vi "Semianalisys.vi"() -> ()   [LabVIEW 2013]
panel:
  in  "?":enum32{"Diode", "BJT", "FET"}(tab)
  out "Voltage versus current curve of diode":cluster{dbl[], dbl[]}(graph)
  out "Ib versus Vbe progress":dbl(slide) scale=0.0..100.0
  in  "R (kOhm)":dbl=1000000.0 format="%#_13g"
  in  "V_AO0 step (V)":dbl=0.01 format="%#_13g"
  in  "OK Button 5":bool
  in  "OK Button":bool
  in  "OK Button 2":bool
  out "Vce versus Ic curve(s)":cluster{"Array":dbl[], dbl[]}(graph)
  out "Ic versus Vce progress":dbl(slide) scale=0.0..100.0
  out "Vbe versus Ib curve":cluster{dbl[], dbl[]}(graph)
  out "Ib versus Vbe progress":dbl(slide) scale=0.0..100.0
  in  "Set several Ib to be plotted on Ic graph (uA)":dbl[](array[numeric])
  in  "Number of curves":i32
  in  "Vce step (V)":dbl=0.1 format="%#_13g"
  in  "R collector (Ohm)":dbl=470.0 format="%#_13g"
  in  "R base (kOhm)":dbl=1000000.0 format="%#_13g"
  in  "Vbe step (V)":dbl=0.01 format="%#_13g"
  in  "Number of curves":i32
  in  "Set several Vgs to be plotted on Vds graph (V)":dbl[](array[numeric])
  in  "Type of FET":u16(ring) items=["JFET", "DMOSFET", "EMOSFET"]
  in  "Vgs step (V)":dbl=0.1 format="%#_13g"
  in  "OK Button 6":bool
  in  "OK Button 7":bool
  in  "R drain (Ohm)":dbl=993.0 format="%#_13g"
  in  "Vds step (V)":dbl=0.1 format="%#_13g"
  out "Id versus Vgs curve":cluster{dbl[], dbl[]}(graph)
  out "Id versus Vgs progress":dbl(slide) scale=0.0..100.0
  out "Id versus Vds curve(s)":cluster{"Array":dbl[], dbl[]}(graph)
  out "Id versus Vds progress":dbl(slide) scale=0.0..100.0
  # "Batyrkhan Saduanov"
  # "Batyrkhan Saduanov"
  # "Batyrkhan Saduanov"
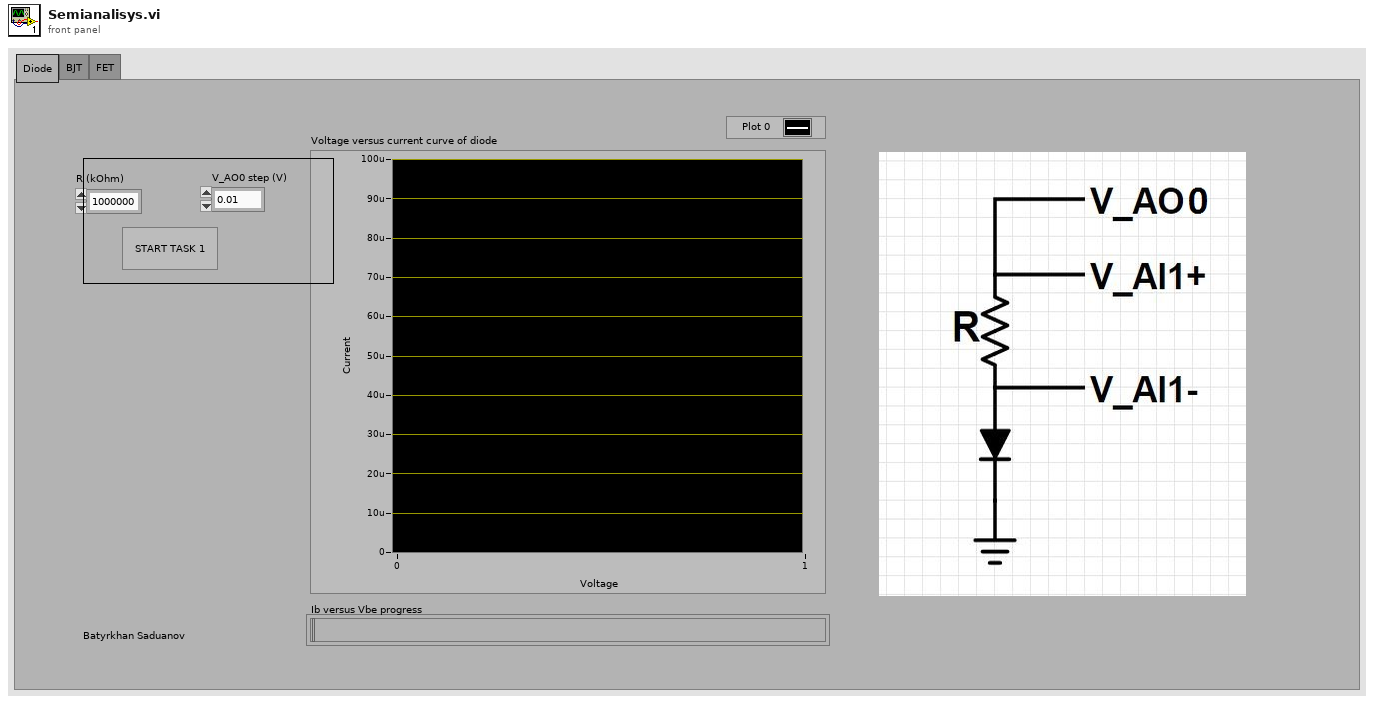
[diagram p1: front panel]
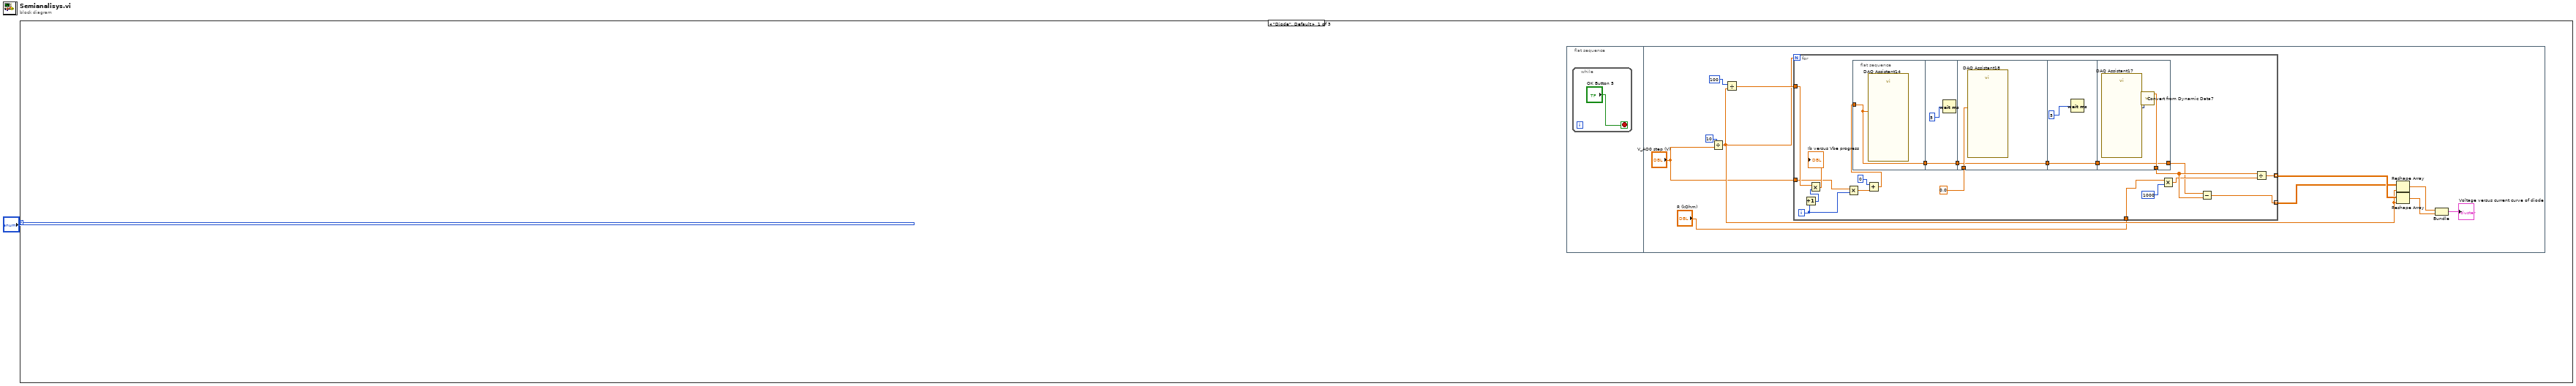
[diagram p0: block diagram]
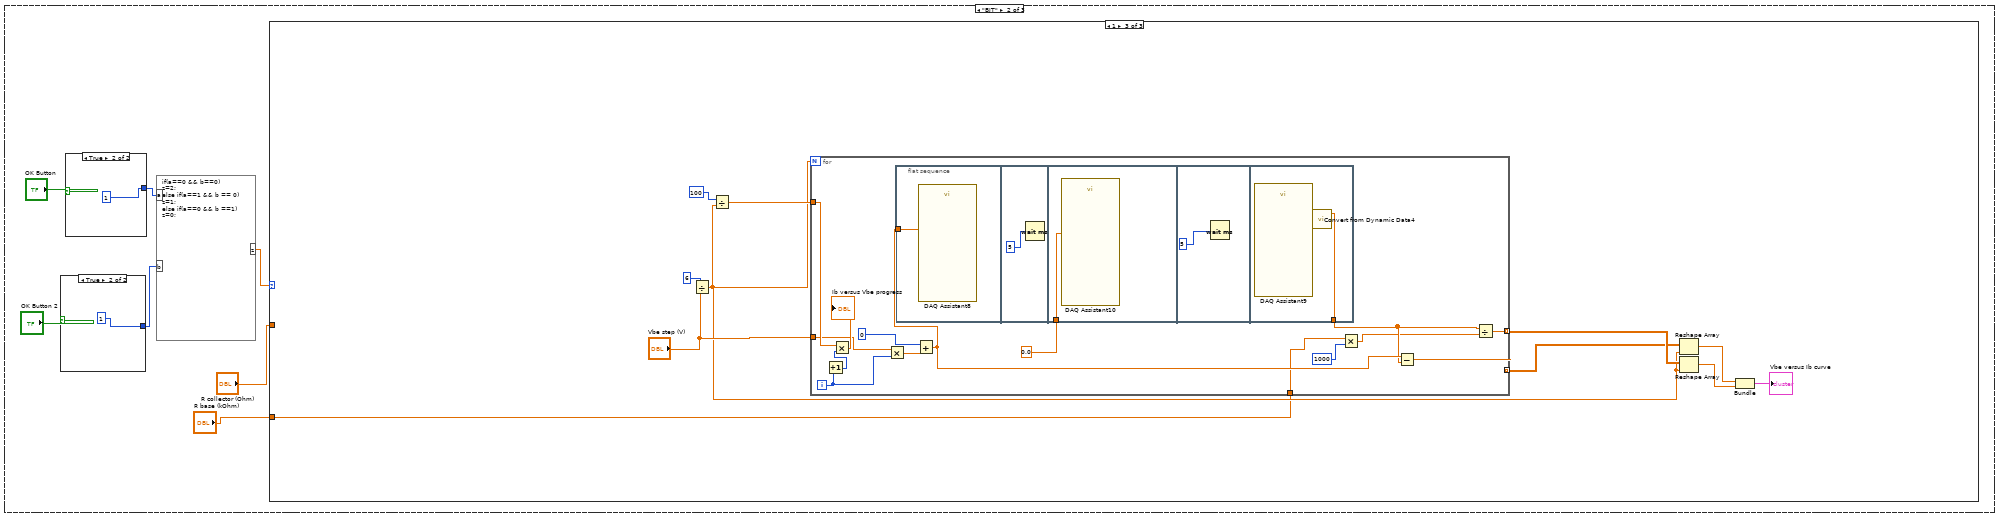
[diagram p2: hidden frame]
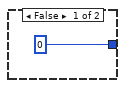
[diagram p3: hidden frame]
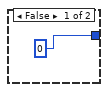
[diagram p4: hidden frame]
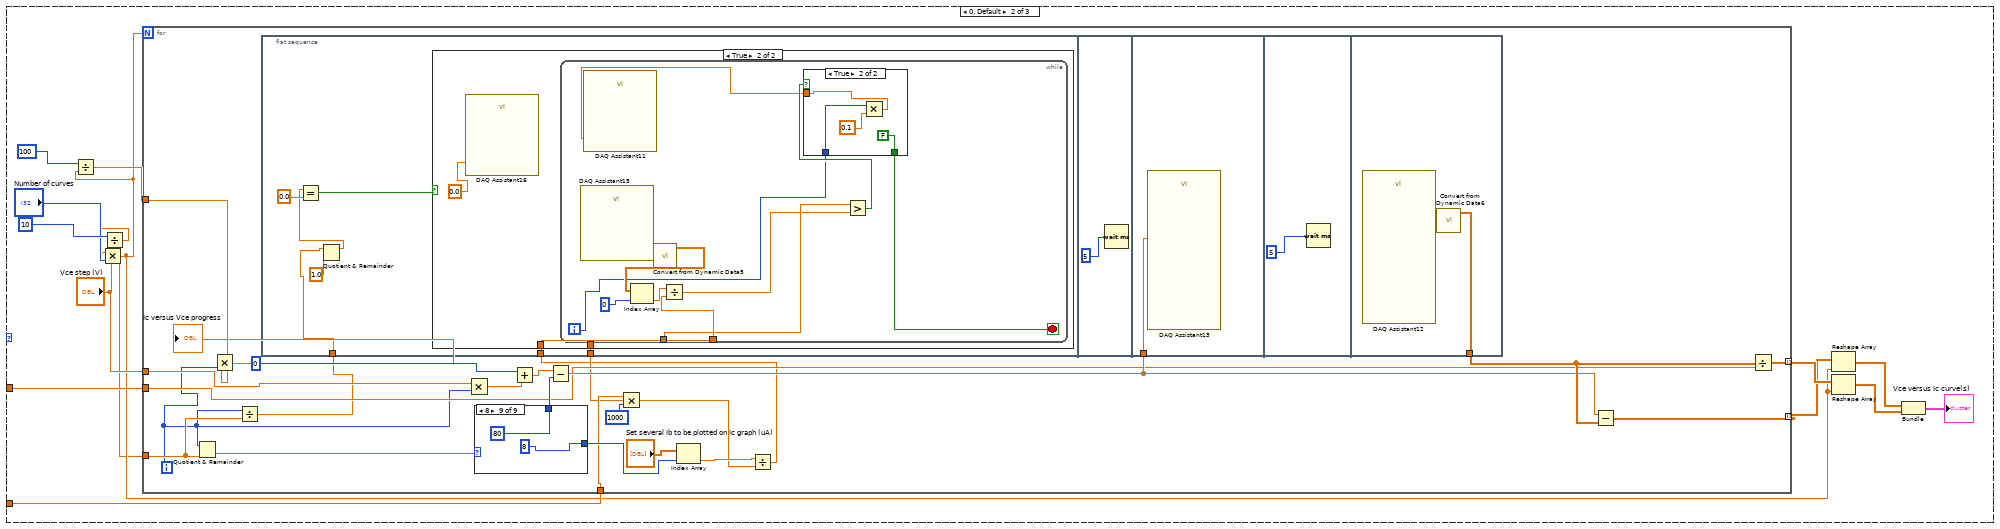
[diagram p6: hidden frame]
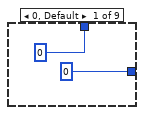
[diagram p7: hidden frame]
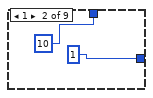
[diagram p8: hidden frame]
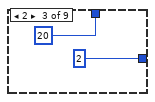
[diagram p9: hidden frame]
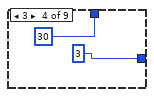
[diagram p10: hidden frame]
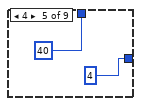
[diagram p11: hidden frame]
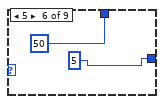
[diagram p12: hidden frame]
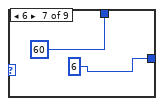
[diagram p13: hidden frame]
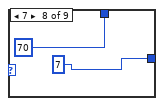
[diagram p14: hidden frame]
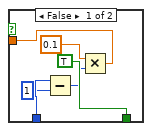
[diagram p16: hidden frame]
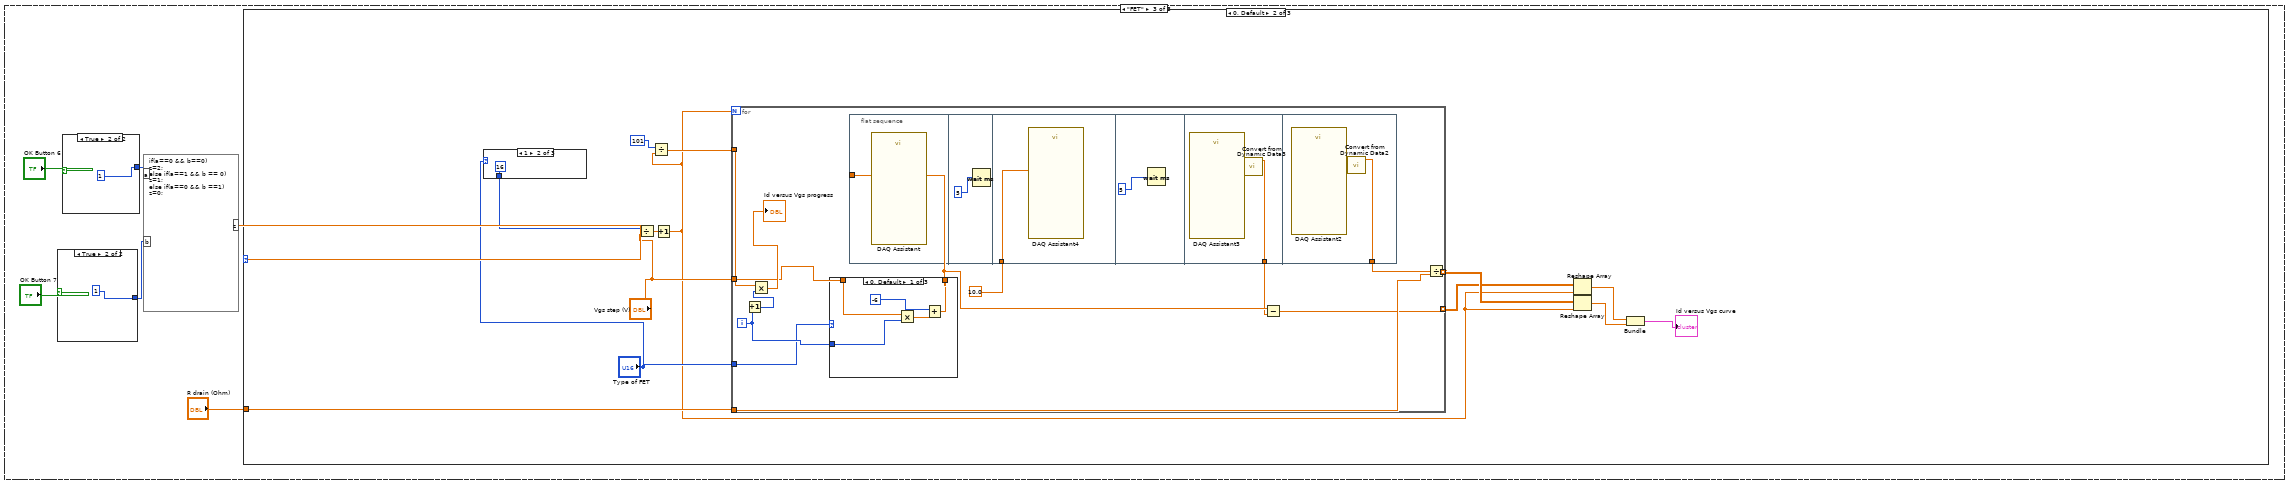
[diagram p17: hidden frame]
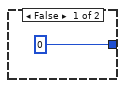
[diagram p18: hidden frame]
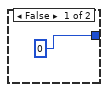
[diagram p19: hidden frame]
diagram:
  n1 = case shown="\"Diode\", Default" "?" {
    frame "Diode", Default {
      n2 = flat-sequence {
        frame #0 {
          n3 = while {
            stop <- "OK Button 5" stop-if-true
          }
        }
        frame #1 {
          n4 = Divide(x=10, y="V_AO0 step (V)") -> (x/y=w5:dbl)
          n5 = Divide(x=100, y=w5) -> (x/y=w9:dbl)
          n6 = for {
            N: w5 -> [_]
            tunnel: [w27] -> w11 mode=indexing
            tunnel: w9 -> [w31]
            tunnel: [w25] -> w7 mode=indexing
            tunnel: "V_AO0 step (V)" -> [w24]
            tunnel: "R (kOhm)" -> [w19]
            i -> [w29]
            n7 = Increment(x=w29) -> (x+1=w28:i32)
            n8 = Multiply(x=w31, y=w28) -> (x*y=→"Ib versus Vbe progress":dbl)
            n9 = Multiply(x=w24, y=w29) -> (x*y=w33:dbl)
            n10 = flat-sequence {
              tunnel: w23 -> [w34]
              tunnel: [w34] -> w14
              tunnel: [w35] -> w15
              tunnel: w14 -> [w35]
              tunnel: 0.0 -> [w38]
              tunnel: [w37] -> w16
              tunnel: w15 -> [w37]
              tunnel: [w39] -> w17
              tunnel: w16 -> [w39]
              tunnel: [w43] -> w22
              tunnel: [w41] -> w18
              tunnel: w17 -> [w41]
              frame #0 {
                n11 = call "DAQ Assistant14"("data"=w34) -> ()  [unwired: 17 in, 2 out]
              }
              frame #1 {
                n12 = Wait (ms)(milliseconds to wait=u32 5) -> ()  [unwired: 1 out]
              }
              frame #2 {
                n13 = call "DAQ Assistant18"("data"=w38) -> ()  [unwired: 17 in, 2 out]
              }
              frame #3 {
                n14 = Wait (ms)(milliseconds to wait=u32 5) -> ()  [unwired: 1 out]
              }
              frame #4 {
                n15 = call "DAQ Assistant17"() -> ("data"=w42:dynamicdata)  [unwired: 17 in, 2 out]
                n16 = call "Convert from Dynamic Data7"("Dynamic Data Type"=w42) -> ("Array"=w43:dbl[])  [unwired: 3 in]
              }
            }
            n17 = Add(x=0, y=w33) -> (x+y=w23:dbl)
            n18 = Multiply(x=w19, y=1000) -> (x*y=w20:dbl)
            n19 = Subtract(x=w18, y=w22) -> (x-y=w25:dbl[])
            n20 = Divide(x=w22, y=w20) -> (x/y=w27:dbl[])
          }
          n21 = Reshape Array(w7, w5) -> (w8:dbl[])
          n22 = Reshape Array(w11, w5) -> (w12:dbl[])
          n23 = Bundle(w8, w12) -> (→"Voltage versus current curve of diode":cluster{dbl[], dbl[]})  [unwired: 1 in]
        }
      }
    }
    frame "BJT" {
      n24 = case shown="True" "OK Button 2" {
        tunnel: [0 1] -> w50
        frame False {
        }
        frame True {
        }
      }
      n25 = case shown="True" "OK Button" {
        tunnel: [0 1] -> w49
        frame False {
        }
        frame True {
        }
      }
      n26 = formula code="if(a==0 && b==0)\nz=2;\nelse if(a==1 && b == 0)\nz=1;\nelse if(a==0 && b ==1)\nz=0;"("a"=w49, "b"=w50) -> ("z"=w46:dbl)
      n27 = case shown="1" w46 {
        tunnel: "R base (kOhm)" -> [_ w62 w146]
        tunnel: "R collector (Ohm)" -> [_ w61 _]
        frame 2 {
        }
        frame 0, Default {
          n28 = Divide(x=10, y="Vce step (V)") -> (x/y=w55:dbl)
          n29 = Multiply(x=w55, y="Number of curves") -> (x*y=w56:dbl)
          n30 = Divide(x=100, y=w56) -> (x/y=w65:dbl)
          n31 = for {
            N: w56 -> [_]
            tunnel: [w87] -> w66 mode=indexing
            tunnel: w65 -> [w89]
            tunnel: [w84] -> w63 mode=indexing
            tunnel: w55 -> [w71]
            tunnel: "Vce step (V)" -> [w80]
            tunnel: w62 -> [w76]
            tunnel: w61 -> [w75]
            i -> [w69]
            n32 = Quotient & Remainder(x=w69, y=w71) -> (floor(x/y)=w81:dbl)  [unwired: 1 out]
            n33 = Multiply(x=w89, y=w69) -> (x*y=→"Ic versus Vce progress":dbl)
            n34 = Divide(x=w69, y=w71) -> (x/y=w70:dbl)
            n35 = flat-sequence {
              tunnel: w73 -> [w116]
              tunnel: w72 -> [w115]
              tunnel: w70 -> [w112]
              tunnel: w79 -> [w142]
              tunnel: [w144] -> w85
              frame #0 {
                n36 = Quotient & Remainder(x=w112, y=1.0) -> (x-y*floor(x/y)=w110:dbl)  [unwired: 1 out]
                n37 = Equal?(x=w110, y=0.0) -> (x = y?=w113:bool)
                n38 = case shown="True" w113 {
                  tunnel: w116 -> [_ w119]
                  tunnel: w115 -> [_ w118]
                  frame False {
                  }
                  frame True {
                    n39 = call "DAQ Assistant16"("data"=0.0) -> ()  [unwired: 17 in, 2 out]
                    n40 = while {
                      tunnel: w119 -> [w127]
                      tunnel: w118 -> [w126]
                      i -> [w121]
                      stop <- w120 stop-if-true
                      n41 = call "DAQ Assistant15"() -> ("data"=w130:dynamicdata)  [unwired: 17 in, 2 out]
                      n42 = call "Convert from Dynamic Data5"("Dynamic Data Type"=w130) -> ("Array"=w128:dbl[])  [unwired: 3 in]
                      n43 = Index Array(array=w128, index=0) -> (element=w122:dbl)
                      n44 = Divide(x=w122, y=w127) -> (x/y=w125:dbl)
                      n45 = Greater?(x=w126, y=w125) -> (0:w124:bool)
                      n46 = case shown="True" w124 {
                        tunnel: [w131 w138] -> w123
                        tunnel: w121 -> [w135 w140]
                        tunnel: [TRUE FALSE] -> w120
                        frame False {
                          n47 = Subtract(x=w135, y=1) -> (x-y=w132:i32)
                          n48 = Multiply(x=0.1, y=w132) -> (x*y=w131:dbl)
                        }
                        frame True {
                          n49 = Multiply(x=w140, y=0.1) -> (x*y=w138:dbl)
                        }
                      }
                      n50 = call "DAQ Assistant11"("data"=w123) -> ()  [unwired: 17 in, 2 out]
                    }
                  }
                }
              }
              frame #1 {
                n51 = Wait (ms)(milliseconds to wait=u32 5) -> ()  [unwired: 1 out]
              }
              frame #2 {
                n52 = call "DAQ Assistant13"("data"=w142) -> ()  [unwired: 17 in, 2 out]
              }
              frame #3 {
                n53 = Wait (ms)(milliseconds to wait=u32 5) -> ()  [unwired: 1 out]
              }
              frame #4 {
                n54 = call "DAQ Assistant12"() -> ("data"=w145:dynamicdata)  [unwired: 17 in, 2 out]
                n55 = call "Convert from Dynamic Data6"("Dynamic Data Type"=w145) -> ("Array"=w144:dbl[])  [unwired: 3 in]
              }
            }
            n56 = Multiply(x=w80, y=w69) -> (x*y=w91:dbl)
            n57 = case shown="8" w81 {
              tunnel: [0 1 2 3 4 5 6 7 8] -> w86
              tunnel: [0 10 20 30 40 50 60 70 80] -> w82
              frame 0, Default {
              }
              frame 1 {
              }
              frame 2 {
              }
              frame 3 {
              }
              frame 4 {
              }
              frame 5 {
              }
              frame 6 {
              }
              frame 7 {
              }
              frame 8 {
              }
            }
            n58 = Add(x=0, y=w91) -> (x+y=w83:dbl)
            n59 = Subtract(x=w83, y=w82) -> (x-y=w79:dbl)
            n60 = Multiply(x=w76, y=1000) -> (x*y=w73:dbl)
            n61 = Index Array(array="Set several Ib to be plotted on Ic graph (uA)", index=w86) -> (element=w74:dbl)
            n62 = Divide(x=w74, y=w73) -> (x/y=w72:dbl)
            n63 = Subtract(x=w79, y=w85) -> (x-y=w84:dbl[])
            n64 = Divide(x=w85, y=w75) -> (x/y=w87:dbl[])
          }
          n65 = Reshape Array(w63, w56) -> (w64:dbl[])
          n66 = Reshape Array(w66, w56) -> (w67:dbl[])
          n67 = Bundle(w64, w67) -> (→"Vce versus Ic curve(s)":cluster{dbl[], dbl[]})  [unwired: 1 in]
        }
        frame 1 {
          n68 = Divide(x=6, y="Vbe step (V)") -> (x/y=w147:dbl)
          n69 = Divide(x=100, y=w147) -> (x/y=w152:dbl)
          n70 = for {
            N: w147 -> [_]
            tunnel: [w165] -> w154 mode=indexing
            tunnel: w152 -> [w169]
            tunnel: [w163] -> w150 mode=indexing
            tunnel: "Vbe step (V)" -> [w162]
            tunnel: w146 -> [w157]
            i -> [w167]
            n71 = Increment(x=w167) -> (x+1=w166:i32)
            n72 = Multiply(x=w169, y=w166) -> (x*y=→"Ib versus Vbe progress":dbl)
            n73 = Multiply(x=w162, y=w167) -> (x*y=w171:dbl)
            n74 = flat-sequence {
              tunnel: w161 -> [w172]
              tunnel: 0.0 -> [w174]
              tunnel: [w177] -> w160
              frame #0 {
                n75 = call "DAQ Assistant8"("data"=w172) -> ()  [unwired: 17 in, 2 out]
              }
              frame #1 {
                n76 = Wait (ms)(milliseconds to wait=u32 5) -> ()  [unwired: 1 out]
              }
              frame #2 {
                n77 = call "DAQ Assistant10"("data"=w174) -> ()  [unwired: 17 in, 2 out]
              }
              frame #3 {
                n78 = Wait (ms)(milliseconds to wait=u32 5) -> ()  [unwired: 1 out]
              }
              frame #4 {
                n79 = call "DAQ Assistant9"() -> ("data"=w176:dynamicdata)  [unwired: 17 in, 2 out]
                n80 = call "Convert from Dynamic Data4"("Dynamic Data Type"=w176) -> ("Array"=w177:dbl[])  [unwired: 3 in]
              }
            }
            n81 = Add(x=0, y=w171) -> (x+y=w161:dbl)
            n82 = Multiply(x=w157, y=1000) -> (x*y=w158:dbl)
            n83 = Subtract(x=w161, y=w160) -> (x-y=w163:dbl[])
            n84 = Divide(x=w160, y=w158) -> (x/y=w165:dbl[])
          }
          n85 = Reshape Array(w150, w147) -> (w151:dbl[])
          n86 = Reshape Array(w154, w147) -> (w155:dbl[])
          n87 = Bundle(w151, w155) -> (→"Vbe versus Ib curve":cluster{dbl[], dbl[]})  [unwired: 1 in]
        }
      }
    }
    frame "FET" {
      n88 = case shown="True" "OK Button 7" {
        tunnel: [0 1] -> w183
        frame False {
        }
        frame True {
        }
      }
      n89 = case shown="True" "OK Button 6" {
        tunnel: [0 1] -> w182
        frame False {
        }
        frame True {
        }
      }
      n90 = formula code="if(a==0 && b==0)\nz=2;\nelse if(a==1 && b == 0)\nz=1;\nelse if(a==0 && b ==1)\nz=0;"("a"=w182, "b"=w183) -> ("z"=w179:dbl)
      n91 = case shown="0, Default" w179 {
        tunnel: "R drain (Ohm)" -> [_ w190 w240]
        frame 2 {
        }
        frame 0, Default {
          n92 = case shown="1" "Type of FET" {
            tunnel: [6 16 10] -> w191
            frame 0, Default {
            }
            frame 1 {
            }
            frame 2 {
            }
          }
          n93 = Divide(x=w191, y="Vgs step (V)") -> (x/y=w189:dbl)
          n94 = Increment(x=w189) -> (x+1=w188:dbl)
          n95 = Divide(x=101, y=w188) -> (x/y=w197:dbl)
          n96 = for {
            N: w188 -> [_]
            tunnel: [w213] -> w199 mode=indexing
            tunnel: w197 -> [w216]
            tunnel: [w204] -> w195 mode=indexing
            tunnel: "Vgs step (V)" -> [w209]
            tunnel: "Type of FET" -> [w208]
            tunnel: w190 -> [w207]
            i -> [w210]
            n97 = Increment(x=w210) -> (x+1=w215:i32)
            n98 = Multiply(x=w216, y=w215) -> (x*y=→"Id versus Vgs progress":dbl)
            n99 = case shown="0, Default" w208 {
              tunnel: [w219 w222 w227] -> w206
              tunnel: w210 -> [w218 w223 w229]
              tunnel: w209 -> [w217 w224 w228]
              frame 0, Default {
                n100 = Multiply(x=w217, y=w218) -> (x*y=w221:dbl)
                n101 = Add(x=-6, y=w221) -> (x+y=w219:dbl)
              }
              frame 1 {
                n102 = Multiply(x=w224, y=w223) -> (x*y=w226:dbl)
                n103 = Add(x=-6, y=w226) -> (x+y=w222:dbl)
              }
              frame 2 {
                n104 = Multiply(x=w228, y=w229) -> (x*y=w230:dbl)
                n105 = Add(x=0, y=w230) -> (x+y=w227:dbl)
              }
            }
            n106 = flat-sequence {
              tunnel: w206 -> [w232]
              tunnel: 10.0 -> [w234]
              tunnel: [w237] -> w205
              tunnel: [w238] -> w214
              frame #0 {
                n107 = call "DAQ Assistant"("data"=w232) -> ()  [unwired: 17 in, 2 out]
              }
              frame #1 {
                n108 = Wait (ms)(milliseconds to wait=u32 5) -> ()  [unwired: 1 out]
              }
              frame #2 {
                n109 = call "DAQ Assistant4"("data"=w234) -> ()  [unwired: 17 in, 2 out]
              }
              frame #3 {
                n110 = Wait (ms)(milliseconds to wait=u32 5) -> ()  [unwired: 1 out]
              }
              frame #4 {
                n111 = call "DAQ Assistant3"() -> ("data"=w236:dynamicdata)  [unwired: 17 in, 2 out]
                n112 = call "Convert from Dynamic Data3"("Dynamic Data Type"=w236) -> ("Array"=w237:dbl[])  [unwired: 3 in]
              }
              frame #5 {
                n113 = call "DAQ Assistant2"() -> ("data"=w239:dynamicdata)  [unwired: 17 in, 2 out]
                n114 = call "Convert from Dynamic Data2"("Dynamic Data Type"=w239) -> ("Array"=w238:dbl[])  [unwired: 3 in]
              }
            }
            n115 = Subtract(x=w206, y=w205) -> (x-y=w204:dbl[])
            n116 = Divide(x=w214, y=w207) -> (x/y=w213:dbl[])
          }
          n117 = Reshape Array(w195, w188) -> (w196:dbl[])
          n118 = Reshape Array(w199, w188) -> (w200:dbl[])
          n119 = Bundle(w196, w200) -> (→"Id versus Vgs curve":cluster{dbl[], dbl[]})  [unwired: 1 in]
        }
        frame 1 {
          n120 = Divide(x=10, y="Vds step (V)") -> (x/y=w241:dbl)
          n121 = Multiply(x="Number of curves", y=w241) -> (x*y=w242:dbl)
          n122 = Divide(x=100, y=w242) -> (x/y=w249:dbl)
          n123 = for {
            N: w242 -> [_]
            tunnel: [w270] -> w251 mode=indexing
            tunnel: w249 -> [w271]
            tunnel: [w265] -> w247 mode=indexing
            tunnel: w241 -> [w269]
            tunnel: "Vds step (V)" -> [w254]
            tunnel: w240 -> [w253]
            i -> [w262]
            n124 = Increment(x=w262) -> (x+1=w261:i32)
            n125 = Multiply(x=w271, y=w261) -> (x*y=→"Id versus Vds progress":dbl)
            n126 = Quotient & Remainder(x=w261, y=w269) -> (floor(x/y)=w260:dbl)  [unwired: 1 out]
            n127 = Multiply(x=w254, y=w262) -> (x*y=w273:dbl)
            n128 = flat-sequence {
              tunnel: w267 -> [w292]
              tunnel: w257 -> [w294]
              tunnel: [w296] -> w266
              frame #0 {
                n129 = call "DAQ Assistant5"("data"=w292) -> ()  [unwired: 17 in, 2 out]
              }
              frame #1 {
                n130 = Wait (ms)(milliseconds to wait=u32 5) -> ()  [unwired: 1 out]
              }
              frame #2 {
                n131 = call "DAQ Assistant7"("data"=w294) -> ()  [unwired: 17 in, 2 out]
              }
              frame #3 {
                n132 = Wait (ms)(milliseconds to wait=u32 5) -> ()  [unwired: 1 out]
              }
              frame #4 {
                n133 = call "DAQ Assistant6"() -> ("data"=w297:dynamicdata)  [unwired: 17 in, 2 out]
                n134 = call "Convert from Dynamic Data"("Dynamic Data Type"=w297) -> ("Array"=w296:dbl[])  [unwired: 3 in]
              }
            }
            n135 = case shown="8" w260 {
              tunnel: [0 1 2 3 4 5 6 7 8] -> w268
              tunnel: [0 10 20 30 40 50 60 70 80] -> w263
              frame 0, Default {
              }
              frame 1 {
              }
              frame 2 {
              }
              frame 3 {
              }
              frame 4 {
              }
              frame 5 {
              }
              frame 6 {
              }
              frame 7 {
              }
              frame 8 {
              }
            }
            n136 = Add(x=0, y=w273) -> (x+y=w264:dbl)
            n137 = Subtract(x=w264, y=w263) -> (x-y=w259:dbl)
            n138 = Subtract(x=w259, y=0.0) -> (x-y=w257:dbl)
            n139 = Index Array(array="Set several Vgs to be plotted on Vds graph (V)", index=w268) -> (element=w267:dbl)
            n140 = Subtract(x=w257, y=w266) -> (x-y=w265:dbl[])
            n141 = Divide(x=w266, y=w253) -> (x/y=w270:dbl[])
          }
          n142 = Reshape Array(w247, w242) -> (w248:dbl[])
          n143 = Reshape Array(w251, w242) -> (w252:dbl[])
          n144 = Bundle(w248, w252) -> (→"Id versus Vds curve(s)":cluster{dbl[], dbl[]})  [unwired: 1 in]
        }
      }
    }
  }
